vi "Update Enable States.vi"(8 "error in (no error)":errorcluster, 10 "ATM State":T1, 11 "ATM View Model in":refnum<class "ATM View Model.lvclass">) -> (0 "error out":errorcluster)   [LabVIEW 2020, in "ATM View Model.lvclass"]
uses:
  ATM View Model.lvclass
  ATM Controller/State.ctl
  ATM View Model.lvclass/ATM View Model.ctl
  ATM Controller/ATM Controller.lvclass
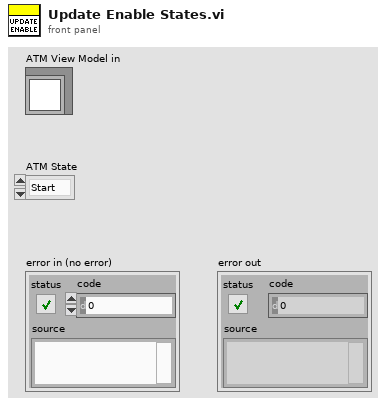
[diagram p1: front panel]
types:
  T1 = typedef "ATM Controller.lvclass/State.ctl" = enum16{"Start", "Card Inserted", "Verification Failed", "Verification Succeeded", "Depositing", "Depositing Completed", "Terminate"}
  T2 = typedef "ATM View Model.lvclass/Controls.ctl" = enum16{"User Input", "Enter", "Left Menu", "Right Menu", "Left Button", "Right Button", "Card Simulator"}
  T3 = enum8{"Enabled", "Disabled", "Disabled and Grayed Out"}
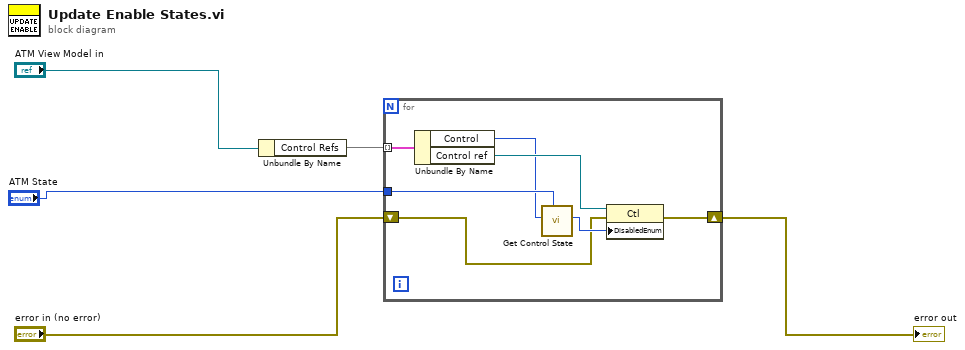
[diagram p0: block diagram]
diagram:
  n1 = Unbundle By Name("ATM View Model in") -> ("Control Refs"=w3:map{T2, refnum<vi>})
  n2 = for {
    tunnel: "ATM State" -> [w12]
    tunnel: w3 -> [w11] mode=indexing
    shift-right: [w6] -> w5
    shift-left: "error in (no error)" -> [w7]
    n3 = Unbundle By Name(w11) -> ("Control"=w8:T2, "Control ref"=w10:refnum<vi>)
    n4 = call "Get Control State.vi"("ATM State"=w12, "Controls"=w8) -> ("Enable State"=w9:T3)  [unwired: 9 in]
    n5 = property class="Ctl"(reference=w10, error in=w7, "DisabledEnum"=w9) -> (error out=w6:errorcluster)  [unwired: 1 out]
  }
  "error out" <- w5
